vi "Send an MCP Image.vi"() -> ()   [LabVIEW 2018]
uses:
  228d909d-41a9-4f79-baed-15af9dfe542c.vi
  228d909d-41a9-4f79-baed-15af9dfe542c.vi/8b8e546f-609c-4909-9c78-7812a036b31c.vi
  <vilib>/Utility/MD5Checksum.llb/MD5Checksum File.vi
  feGEM DataPacker.lvlib
panel:
  in  "File":path
  in  "?":bool
  in  "MIDAS Sever Port":u16=12345
  in  "MIDAS Server":string="my_midas_server.domain"
  out "Files Sent":i32
  in  "Click button to send file":bool
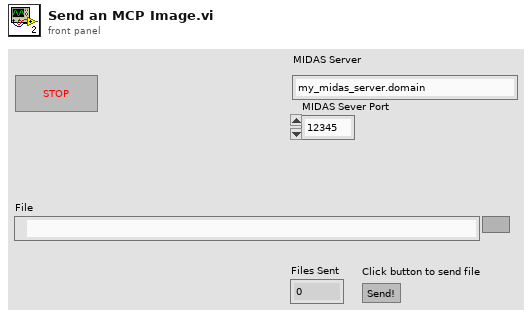
[diagram p1: front panel]
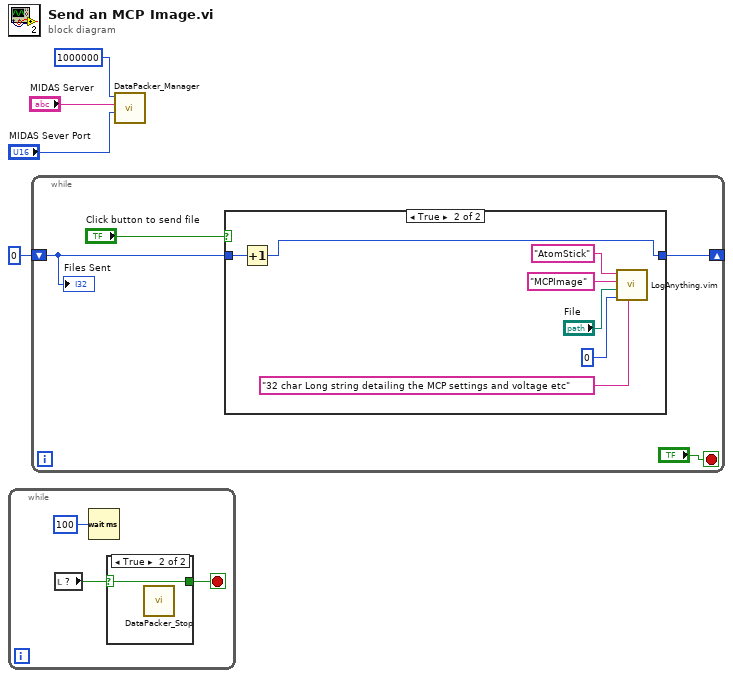
[diagram p0: block diagram]
diagram:
  n1 = while {
    stop <- w6 stop-if-true
    n2 = local read item#4() -> (w5:bool)
    n3 = Wait (ms)(milliseconds to wait=u32 100) -> ()  [unwired: 1 out]
    n4 = case shown="True" w5 {
      selector: w5 -> [w8 w9]
      tunnel: [w8 w9] -> w6
      frame False {
      }
      frame True {
        n5 = call "DataPacker_Stop.vi"() -> ()  [unwired: 12 in]
      }
    }
  }
  n6 = while {
    shift-right: [w11] -> _
    shift-left: 0 -> [w12]
    stop <- "?" stop-if-true
    n7 = case shown="True" "Click button to send file" {
      tunnel: w12 -> [w14 w21]
      tunnel: [w14 w20] -> w11
      frame False {
      }
      frame True {
        n8 = Increment(x=w21) -> (x+1=w20:i32)
        n9 = call "LogAnything.vim"("Equipment description (32 chars)"="32 char Long string detailing the MCP settings and voltage etc" ("Project Name (Unlimited length... Key word for analyzer, or folder for MIDAS settings file database)"), "Period to update history plots (seconds)\nUnset (65535) = Use MIDAS default in ODB\n0 = Record but do not put in histories"=u16 0 ("Period to update history plots (seconds)\nUnset (65535) = Use MIDAS default in ODB\n0 = Record but do not put in histories"), "Array"="File", "Variable Name"="MCPImage" ("Variable name (SAVE and LOAD are magic keywords for the MIDAS settings file database)"), "Category"="AtomStick" ("Category (SETTINGS_FILE is a magic keyword for the MIDAS settings file database)")) -> ()  [unwired: 6 in, 1 out]
      }
    }
    "Files Sent" <- w12
  }
  n10 = call "DataPacker_Manager.vi"("MIDAS Sever Port"="MIDAS Sever Port", "MIDAS Server"="MIDAS Server", "Override Max Event size (Data rate bytes/s). Use MIDAS Default = 0"=u32 1000000 ("Override Max Event size (Data rate kb/s). Use MIDAS Default = 0")) -> ()  [unwired: 9 in]
